vi "load_from_file.vi"() -> ()   [LabVIEW 2016]
uses:
  <vilib>/Utility/file.llb/Read Delimited Spreadsheet (DBL).vi
panel:
  in  "# hidden layers":i32=1
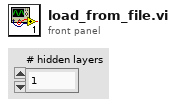
[diagram p1: front panel]
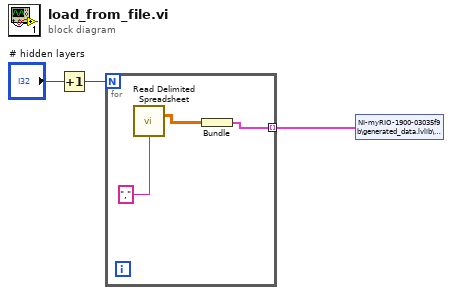
[diagram p0: block diagram]
diagram:
  n1 = Increment(x="# hidden layers") -> (x+1=w1:i32)
  n2 = for {
    N: w1 -> [_]
    tunnel: [w4] -> w3 mode=indexing
    n3 = call-poly <vilib>:"Read Delimited Spreadsheet.vi"("delimiter (\\t)"=",") -> ("all rows"=w6:dbl[][])  [unwired: 9 in, 5 out]
    n4 = Bundle("all rows"=w6) -> (w4:cluster{"all rows":dbl[][]})  [unwired: 1 in]
  }
  n5 = shared-variable "NI-myRIO-1900-03035f9b\\generated_data.lvlib\\Weights"(w3) -> ()  [unwired: 1 in, 1 out]
